vi "Create Log File.vi"(8 "error in (no error)":errorcluster, 11 "Message Log in":refnum<class "Message Log.lvclass">) -> (0 "error out":errorcluster, 3 "Message Log out":refnum<class "Message Log.lvclass">)   [LabVIEW 2017, in "Message Log.lvclass"]
doc: "Create Log File if it has not yet been created"
uses:
  Message Log.lvclass
  Message Log.lvclass/Message Log.ctl
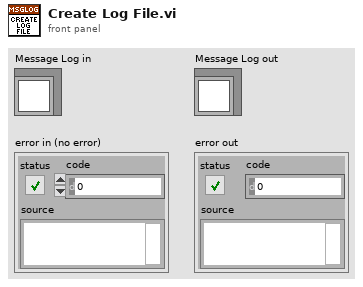
[diagram p1: front panel]
types:
  T1 = enum16{"open", "replace", "create", "open or create", "replace or create", "replace or create with confirmation"}
  T2 = typedef "Message Log ID.ctl" = cluster{"Head Worker ID":string, "IP Address":string}
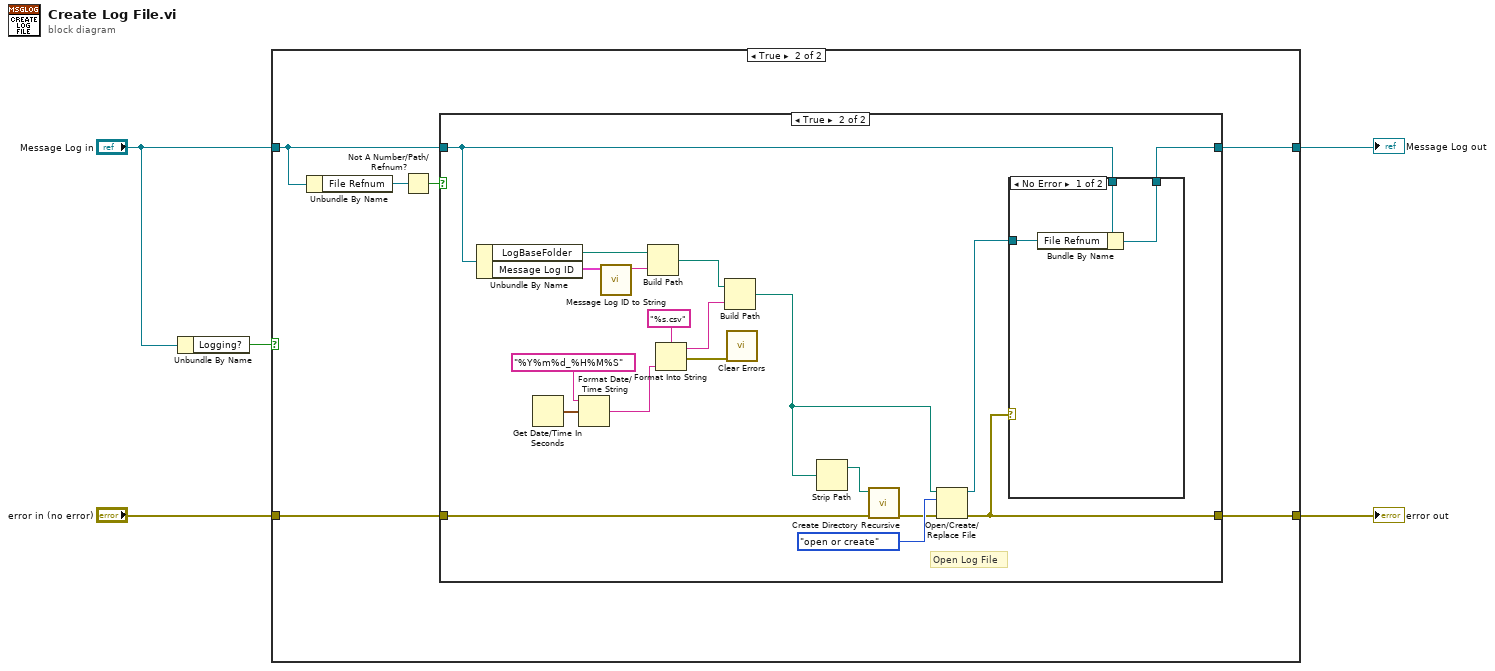
[diagram p0: block diagram]
diagram:
  n1 = Unbundle By Name("Message Log in") -> ("Logging?"=w1:bool)
  n2 = case shown="True" w1 {
    tunnel: [w7 w11] -> w5
    tunnel: "Message Log in" -> [w7 w10]
    tunnel: "error in (no error)" -> [w6 w9]
    tunnel: [w6 w8] -> w3
    frame False {
    }
    frame True {
      n3 = Unbundle By Name(w10) -> ("File Refnum"=w12:refnum<file>)
      n4 = Not A Number/Path/Refnum?(number/path/refnum=w12) -> (NaN/Path/Refnum?=w13:bool)
      n5 = case shown="True" w13 {
        tunnel: [w15 w29] -> w11
        tunnel: w10 -> [w15 w20]
        tunnel: [w14 w28] -> w8
        tunnel: w9 -> [w14 w28]
        frame False {
          # "Log file already created. do nothing"
        }
        frame True {
          # "Open Log File"
          n6 = Unbundle By Name(w20) -> ("LogBaseFolder"=w17:path, "Message Log ID"=w19:T2)
          n7 = Get Date/Time In Seconds() -> (seconds since 1Jan1904=w23:timestamp)
          n8 = Format Date/Time String(time format string (%c)="%Y%m%d_%H%M%S", seconds (now)=w23) -> (date/time string=w22:string)  [unwired: 1 out]
          n9 = call "Message Log ID to String.vi"("Message Log ID"=w19) -> ("Message Log ID String"=w18:string)  [unwired: 10 in]
          n10 = Build Path(base path=w17, name or relative path=w18) -> (appended path=w16:path)
          n11 = Format Into String(format string="%s.csv", w22) -> (resulting string=w26:string, error out=w25:errorcluster)  [unwired: 2 in]
          n12 = Build Path(base path=w16, name or relative path=w26) -> (appended path=w21:path)
          n13 = call <vilib>:"Clear Errors.vi"("error in (no error)"=w25) -> ()  [unwired: 5 in, 2 out]
          n14 = Strip Path(path=w21) -> (stripped path=w32:path)  [unwired: 1 out]
          n15 = call <vilib>:"Create Directory Recursive.vi"("directory"=w32) -> ("error out"=w30:errorcluster)  [unwired: 4 in, 2 out]
          n16 = Open/Create/Replace File(file path (use dialog)=w21, error in=w30, operation (0:open)=T1."open or create") -> (refnum out=w33:refnum<file>)  [unwired: 2 in, 3 out]
          n17 = case shown="No Error" w28 {
            tunnel: w33 -> [w34 _]
            tunnel: w20 -> [w36 w37]
            tunnel: [w35 w37] -> w29
            frame No Error {
              n18 = Bundle By Name(cluster=w36, "File Refnum"=w34) -> (w35:refnum<class "Message Log.lvclass">)
            }
            frame Error {
            }
          }
        }
      }
    }
  }
  "Message Log out" <- w5
  "error out" <- w3
